vi "RichToFlatgrpcservice_AkipResponse.vi"(5 "OutputClusterType":T1, 11 "InputCluster":T2) -> (3 "OutputCluster":T1)   [LabVIEW 2023, in "Proto_client.lvlib"]
uses:
  grpcservice_AkipResponse.ctl
  grpcservice_AkipResponse_Flat.ctl
  Proto_client.lvlib
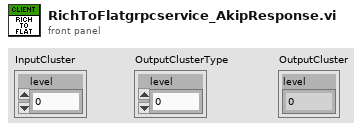
[diagram p1: front panel]
types:
  T1 = typedef "Proto_client.lvlib/grpcservice_AkipResponse_Flat.ctl" = cluster{"level":sgl}
  T2 = typedef "Proto_client.lvlib/grpcservice_AkipResponse.ctl" = cluster{"level":sgl}
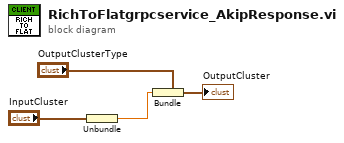
[diagram p0: block diagram]
diagram:
  n1 = Unbundle "Unbundle"("InputCluster") -> ("level"=w1:sgl)
  n2 = Bundle "Bundle"(cluster="OutputClusterType", "level"=w1) -> (→"OutputCluster":T1)
